vi "SaveOnMP.vi"(9 "Contents":string, 10 "File Name":string, 11 "Queue in":refnum<queue>) -> ()   [LabVIEW 2019]
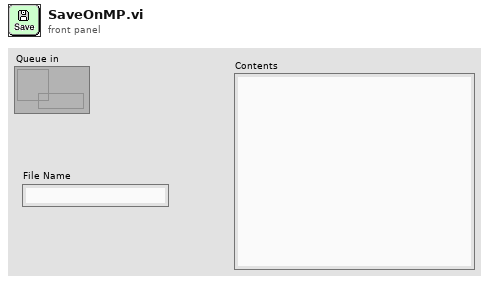
[diagram p1: front panel]
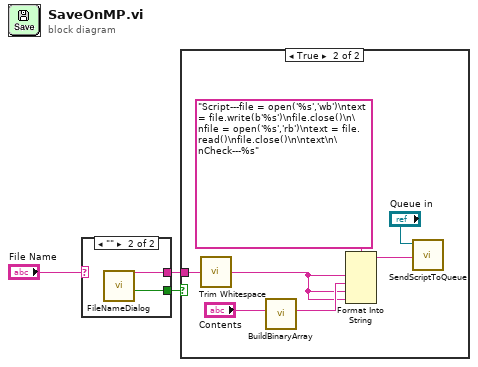
[diagram p0: block diagram]
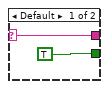
[diagram p3: hidden frame]
diagram:
  n1 = case shown="\"\"" "File Name" {
    selector: "File Name" -> [w5 _]
    tunnel: [w5 w6] -> w1
    tunnel: [TRUE ("OK") w7] -> w2
    frame Default {
    }
    frame "" {
      n2 = call <userlib>:"FileNameDialog.vi"() -> ("OK?"=w7:bool, "String Out"=w6:string)  [unwired: 10 in]
    }
  }
  n3 = case shown="True" w2 {
    tunnel: w1 -> [_ w11]
    frame False {
    }
    frame True {
      n4 = call <vilib>:"Trim Whitespace.vi"("string"=w11) -> ("trimmed string"=w8:string)  [unwired: 1 in]
      n5 = call <userlib>:"BuildBinaryArray.vi"("String in"="Contents") -> ("Binary String out"=w9:string)  [unwired: 10 in]
      n6 = Format Into String(format string="Script---file = open('%s','wb')\ntext = file.write(b'%s')\nfile.close()\n\nfile = open('%s','rb')\ntext = file.read()\nfile.close()\n\ntext\n\nCheck---%s" ("write buffer"), w8, w9, w8, w8) -> (resulting string=w12:string)  [unwired: 2 in, 1 out]
      n7 = call <userlib>:"SendScriptToQueue.vi"("String"=w12, "Queue in"="Queue in") -> ()  [unwired: 10 in]
    }
  }
